vi "initialize.vi"(0 "HGF_SV.lvlib:HGF_SVService.lvclass":refnum<class "HGF_SVService.lvclass">, 3 "initializationData":variant, 5 "error in (no error)":errorcluster, 7 "binaryString":string, 8 "I8 Array":i8[](array[numeric]), 9 "prependSize? (T)":bool, 11 "byteOrder (0:big-endian, network order)":T1(ring)) -> (14 "dup HGF_SV.lvlib:HGF_SVService.lvclass":refnum<class "HGF_SVService.lvclass">, 17 "found?":bool, 19 "error out":errorcluster)   [LabVIEW 2012, in "HGF_SV.lvlib" / "HGF_SVService.lvclass"]
uses:
  HGF_SVService.lvclass
  HGF_BaseClasses/HGF_PVPublisher/HGF_PVPublisher.lvclass
  HGF_SVService.lvclass/HGF_SVService.ctl
  HGF_SV.lvlib
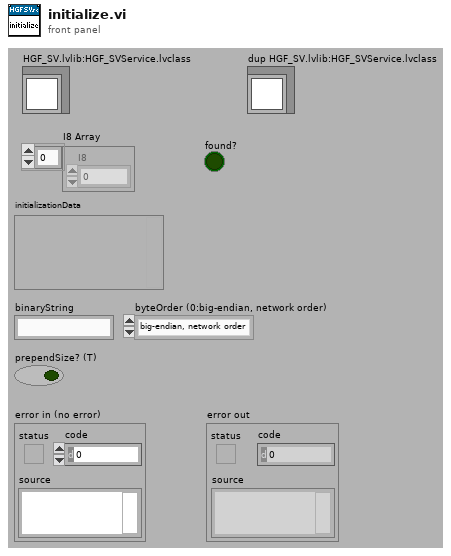
[diagram p1: front panel]
types:
  T1 = enum16{"big-endian, network order", "native, host order", "little-endian"}
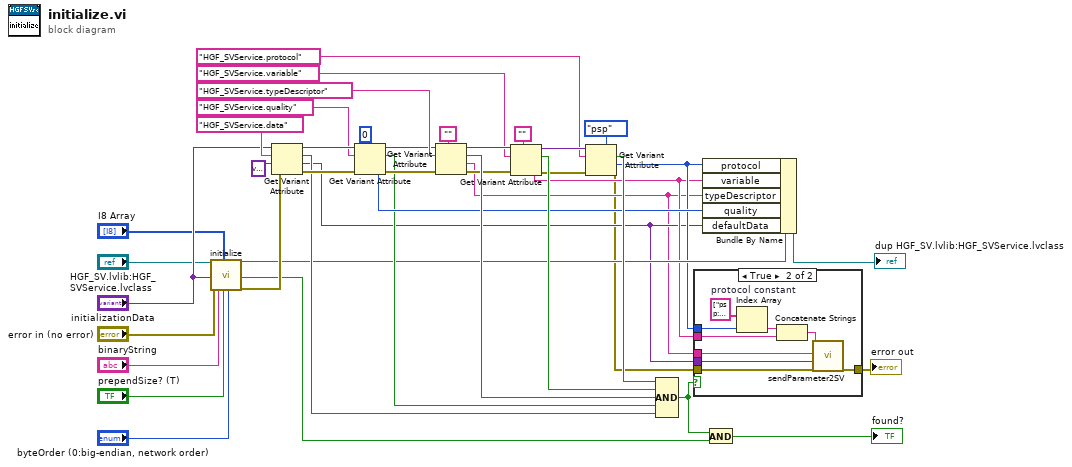
[diagram p0: block diagram]
diagram:
  n1 = call-parent "initialize.vi"("HGV_PVBase"="HGF_SV.lvlib:HGF_SVService.lvclass", "initializationData"="initializationData", "error in (no error)"="error in (no error)", "binaryString"="binaryString", "I8 Array"="I8 Array", "prependSize? (T)"="prependSize? (T)", "byteOrder (0:big-endian, network order)"="byteOrder (0:big-endian, network order)") -> ("HGV_PVBase"=w20:refnum<class "HGF_SVService.lvclass">, "found?"=w2:bool, "error out"=w32:errorcluster)  [unwired: 10 out]
  n2 = Get Variant Attribute(Variant="initializationData", name="HGF_SVService.data", default value (empty Variant)=variant ("initializationData"), error in=w32) -> (duplicate Variant=w35:variant, found=w31:bool, value=w7:variant, error out=w36:errorcluster)
  n3 = Get Variant Attribute(Variant=w35, name="HGF_SVService.quality", default value (empty Variant)=0 ("quality"), error in=w36) -> (duplicate Variant=w37:variant, found=w30:bool, value=w33:i32, error out=w38:errorcluster)
  n4 = Get Variant Attribute(Variant=w37, name="HGF_SVService.typeDescriptor", default value (empty Variant)="", error in=w38) -> (duplicate Variant=w19:variant, found=w41:bool, value=w6:string, error out=w14:errorcluster)
  n5 = Get Variant Attribute(Variant=w19, name="HGF_SVService.variable", default value (empty Variant)="", error in=w14) -> (duplicate Variant=w18:variant, found=w42:bool, value=w10:string, error out=w12:errorcluster)
  n6 = Get Variant Attribute(Variant=w18, name="HGF_SVService.protocol", default value (empty Variant)=enum8{"psp", "opc"}."psp" ("protocol"), error in=w12) -> (found=w43:bool, value=w11:enum8{"psp", "opc"}, error out=w5:errorcluster)  [unwired: 1 out]
  n7 = Compound Arithmetic op=AND(w43, w42, w41, w30, w31) -> (w1:bool)
  n8 = case shown="True" w1 {
    tunnel: w11 -> [_ w52]
    tunnel: w10 -> [_ w50]
    tunnel: w7 -> [_ w48]
    tunnel: w6 -> [_ w47]
    tunnel: w5 -> [w44 w46]
    tunnel: [w44 w45] -> w4
    frame False {
    }
    frame True {
      w53 = string[] ["psp:", "opc:"]  # protocol constant
      n9 = Index Array(array=w53, index=w52) -> (element=w51:string)
      n10 = Concatenate Strings(w51, w50) -> (w49:string)
      n11 = call "sendParameter2SV.vi"("Connection In"=w49, "Parameter"=w48, "typeDescriptor"=w47, "error in (no error)"=w46) -> ("error out"=w45:errorcluster)  [unwired: 1 in, 14 out]
    }
  }
  "error out" <- w4
  n12 = Bundle By Name(cluster=w20, "protocol"=w11, "variable"=w10, "typeDescriptor"=w6, "quality"=w33, "defaultData"=w7) -> (→"dup HGF_SV.lvlib:HGF_SVService.lvclass":refnum<class "HGF_SVService.lvclass">)
  n13 = And(x=w1, y=w2) -> (x .and. y?=→"found?":bool)
